vi "Import Custom SCP Commands List.vi"(8 "error in (no error)":errorcluster, 11 "Node Ptr":u64 format="%.0x") -> (0 "error out":errorcluster)   [LabVIEW 2018, in "Vires VTD System Explorer.lvlib"]
uses:
  Vires VTD System Explorer.lvlib
  <vilib>/Utility/file.llb/Read Delimited Spreadsheet (string).vi
  <vilib>/NI Veristand/Custom Device Tools/Custom Device Utility Library/Custom Device Utility Library.lvlib
panel:
  in  "Tag":string
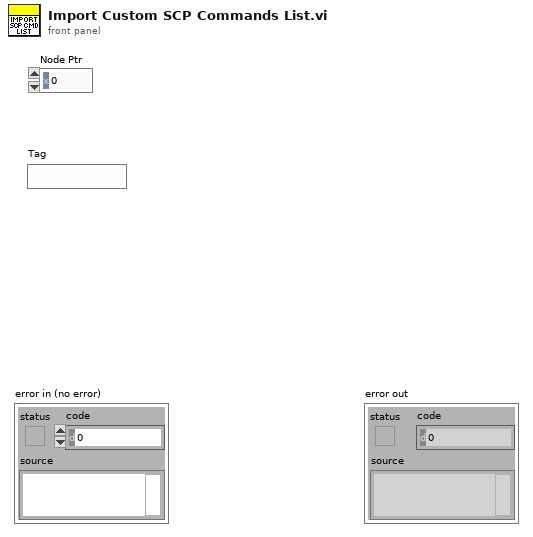
[diagram p1: front panel]
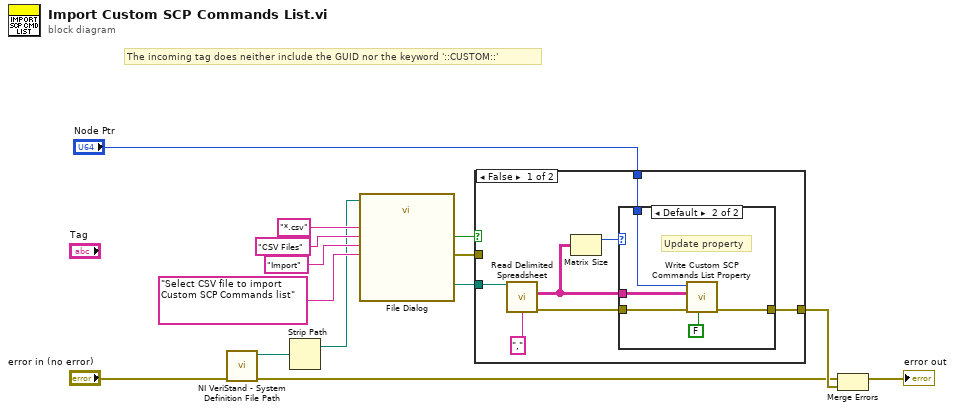
[diagram p0: block diagram]
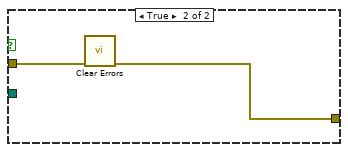
[diagram p3: hidden frame]
diagram:
  # "The incoming tag does neither include the GUID nor the keyword '::CUSTOM::'"
  n1 = call <vilib>:"NI VeriStand - System Definition File Path.vi"("error in (no error)"="error in (no error)") -> ("error out"=w5:errorcluster, "SDF path"=w6:path)  [unwired: 9 in]
  n2 = Strip Path(path=w6) -> (stripped path=w4:path)  [unwired: 1 out]
  n3 = call "File Dialog"("start path"=w4, "prompt"="Select CSV file to import Custom SCP Commands list", "button label"="Import", "pattern (all files)"="*.csv", "pattern label"="CSV Files") -> ("selected path"=w9:path, "cancelled"=w10:bool, "error out"=w8:errorcluster)  [unwired: 7 in, 1 out]
  n4 = case shown="False" w10 {
    tunnel: w9 -> [w21 _]
    tunnel: w8 -> [_ w29]
    tunnel: [w19 w28] -> w7
    tunnel: "Node Ptr" -> [w18 _]
    frame False {
      n5 = call-poly <vilib>:"Read Delimited Spreadsheet.vi"("file path (dialog if empty)"=w21, "delimiter (\\t)"="," ("delimiter (\\t)")) -> ("all rows"=w17:string[][], "error out"=w20:errorcluster)  [unwired: 8 in, 4 out]
      n6 = Matrix Size(0:w17) -> (1:w16:i32)  [unwired: 1 out]
      n7 = case shown="Default" w16 {
        tunnel: w20 -> [w22 w27]
        tunnel: [w22 w26] -> w19
        tunnel: w18 -> [_ w25]
        tunnel: w17 -> [_ w24]
        frame 0 {
          # "no records found\n(Empty CSV?)\n>> do nothing"
        }
        frame Default {
          # "Update property"
          n8 = call "Write Custom SCP Commands List Property.vi"("Remove 1st Column? (T)"=FALSE, "error in (no error)"=w27, "Custom SCP Commands List"=w24, "Node Ptr"=w25) -> ("error out"=w26:errorcluster)  [unwired: 6 in, 1 out]
        }
      }
    }
    frame True {
      n9 = call <vilib>:"Clear Errors.vi"("error in (no error)"=w29) -> ("error out"=w28:errorcluster)  [unwired: 5 in, 1 out]
    }
  }
  n10 = Merge Errors(w5, w7) -> (→"error out":errorcluster)
